vi "PH_Beamline.set Switch+6P State in GUI.vi"(0 "i ref in":refnum<vi>, 1 "Boolean GUI Ref":refnum<vi>, 2 "Picture GUI Ref":refnum<vi>, 3 "Subscriber State":T1 items=["no info", "off/false/out", "on/true/in", "Failure", "Alarm", "Status 1", "Status 2", "Status 3"], 5 "error in (no error)":errorcluster) -> (14 "i ref out":refnum<vi>, 19 "error out":errorcluster)   [LabVIEW 2014, in "PH_Beamline.lvlib"]
doc: "This VI writes the incoming information about a combined switch and 6P to the GUI."
uses:
  PH_Beamline.lvlib
  PH_StatusHandler/PH_StatusHandler.Status.ctl
  PH_Beamline_Common/PH_Beamline_Common.lvlib
  CSCore/CSSystem/CSSystemLib/CSSystemLib.lvlib
  PH_StatusHandler/PH_StatusHandler.lvlib
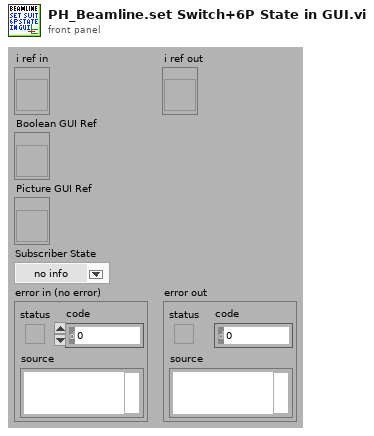
[diagram p1: front panel]
types:
  T1 = typedef "PH_StatusHandler.lvlib/PH_StatusHandler.Status.ctl" = i16
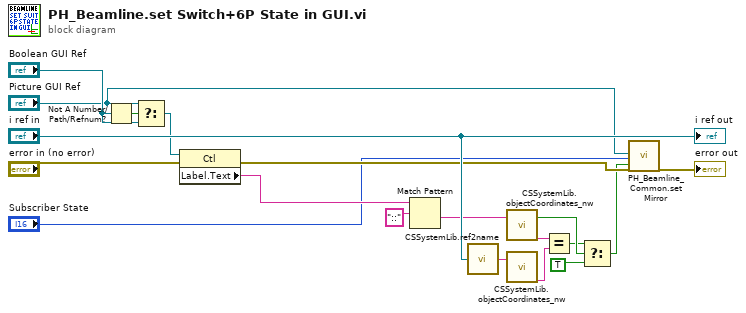
[diagram p0: block diagram]
diagram:
  n1 = Not A Number/Path/Refnum?(number/path/refnum="Boolean GUI Ref") -> (NaN/Path/Refnum?=w16:bool)
  n2 = Select(t="Picture GUI Ref", s=w16, f="Boolean GUI Ref") -> (s? t:f=w17:refnum<vi>)
  n3 = property class="Ctl"(reference=w17, error in="error in (no error)") -> (error out=w14:errorcluster, "Label.Text"=w13:string)  [unwired: 1 out]
  n4 = Match Pattern(string=w13, regular expression="::") -> (after substring=w4:string)  [unwired: 1 in, 3 out]
  n5 = call "CSSystemLib.ref2name.vi"("obj refnum"="i ref in") -> ("name"=w9:string)
  n6 = call "CSSystemLib.objectCoordinates_nw.vi"("name"=w4) -> ("obj exists"=w5:bool, "node"=w6:string)  [unwired: 15 in, 2 out]
  n7 = call "CSSystemLib.objectCoordinates_nw.vi"("name"=w9) -> ("node"=w7:string)  [unwired: 15 in, 3 out]
  n8 = Equal?(x=w6, y=w7) -> (x = y?=w3:bool)
  n9 = Select(t=w3, s=w5, f=TRUE) -> (s? t:f=w2:bool)
  n10 = call "PH_Beamline_Common.set Mirror.vi"("CtlRef"="Picture GUI Ref", "Status (on/true/in)"="Subscriber State", "GUI Instance does not exist or here?"=w2, "error in (no error)"=w14) -> ("error out"=→"error out":errorcluster)  [unwired: 15 in]
  "i ref out" <- "i ref in"
